vi "Get frame.vi"(5 "frame y size":u16, 7 "frame x size":u16, 8 "error in (no error)":errorcluster, 10 "Image in":T1, 11 "camera handle in":i16) -> (0 "error out":errorcluster, 2 "Image out":T1, 3 "camera handle out":i16)   [LabVIEW 2012]
uses:
  <vilib>/vision/Image Controls.llb/IMAQ Image.ctl
  Visual Studio/Cascade wrapper/Release/Cascade wrapper.dll
panel:
  out "min value":u16
  out "max value":u16
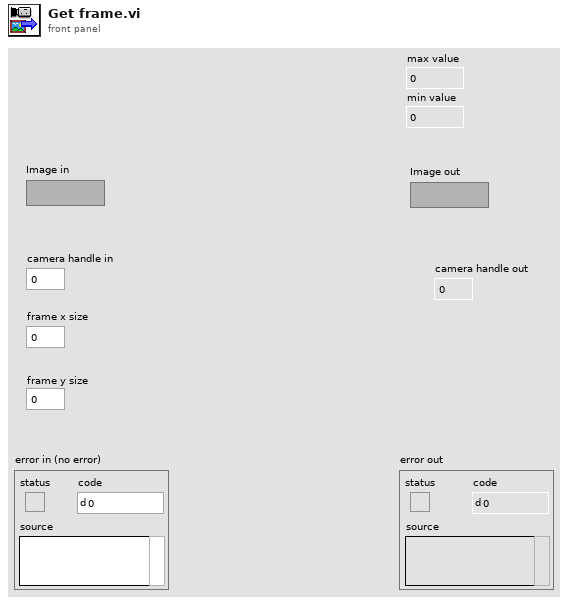
[diagram p1: front panel]
types:
  T1 = typedef "IMAQ Image.ctl" = refnum<image>
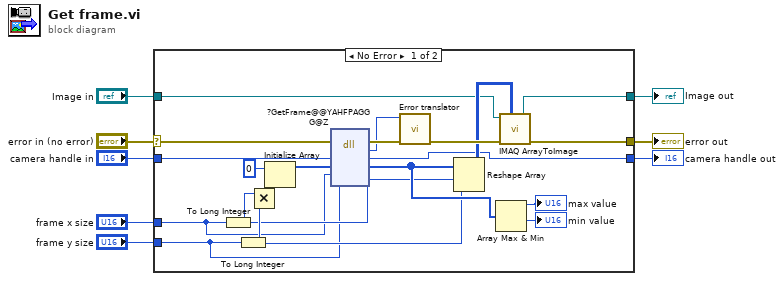
[diagram p0: block diagram]
diagram:
  n1 = case shown="No Error" "error in (no error)" {
    selector: "error in (no error)" -> [w28 w30]
    tunnel: "camera handle in" -> [w27 w29]
    tunnel: "frame x size" -> [w9 _]
    tunnel: "frame y size" -> [w10 _]
    tunnel: "Image in" -> [w22 w31]
    tunnel: [w21 w31] -> w3
    tunnel: [w20 w30] -> w2
    tunnel: [w19 w29] -> w1
    frame No Error {
      n2 = To Long Integer(number=w9) -> (32bit integer=w11:i32)
      n3 = To Long Integer(number=w10) -> (32bit integer=w13:i32)
      n4 = Multiply(x=w11, y=w13) -> (x*y=w12:i32)
      n5 = Initialize Array(u16 0 ("element"), w12) -> (w14:u16[])
      n6 = dll-call lib="C:/moroder/Cascade wrapper/Visual Studio/Cascade wrapper/Release/Cascade wrapper.dll" fn="?GetFrame@@YAHFPAGGG@Z"(error in=w28, "camera handle"=w27, "frame"=w14, "x size"=w9, "y size"=w10) -> (error out=w26:errorcluster, "error"=w25:i32, "camera handle"=w19:i16, "frame"=w16:u16[])  [unwired: 4 in, 1 out]
      n7 = call "Error translator.vi"("error in (no error)"=w26, "error code"=w25) -> ("error out"=w24:errorcluster)  [unwired: 9 in]
      n8 = Reshape Array(w16, w11, w13) -> (w23:u16[][])
      n9 = Array Max & Min(array=w16) -> (max value=→"max value":u16, min value=→"min value":u16)  [unwired: 2 out]
      n10 = call "IMAQ ArrayToImage"("Image Pixels (U16)"=w23, "error in (no error)"=w24, "Image"=w22) -> ("error out"=w20:errorcluster, "Image Out"=w21:T1)  [unwired: 7 in]
    }
    frame Error {
    }
  }
  "error out" <- w2
  "camera handle out" <- w1
  "Image out" <- w3
